vi "UpdateFeatureStudio.vi"(0 "Device In":T1, 5 "FeatureScript":string, 11 "error in":errorcluster) -> (4 "Device Out":T1, 6 "Comm":T2, 15 "error out":errorcluster)   [LabVIEW 2019]
uses:
  <userlib>/IoT Devices/_subVIs/HTTPComm.ctl
  <userlib>/Onshape/_SubVI/Cluster.ctl
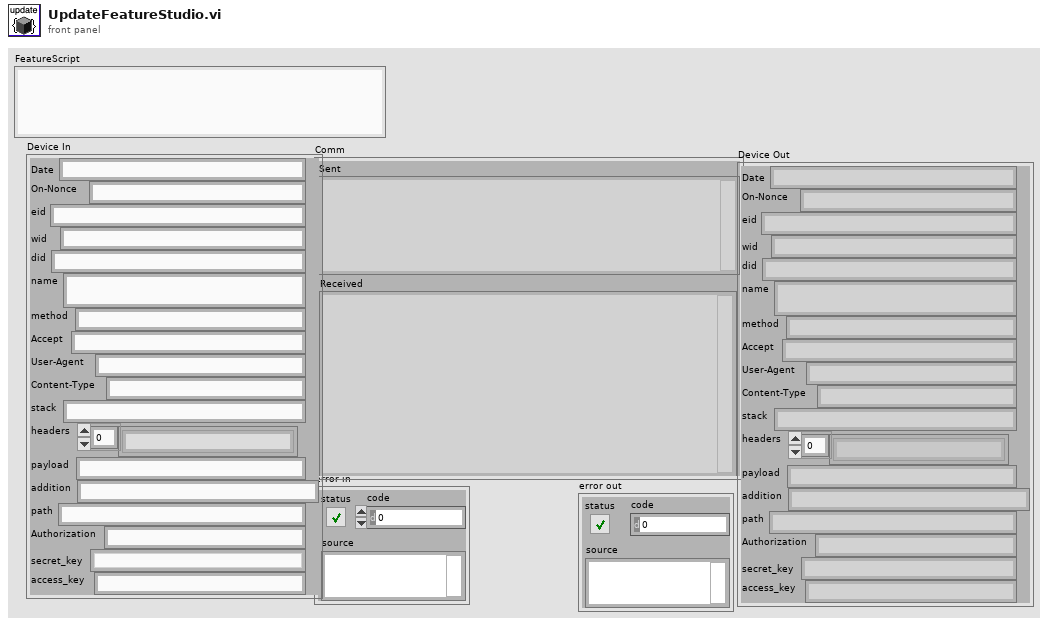
[diagram p1: front panel]
types:
  T1 = typedef "Cluster.ctl" = cluster{"Date":string, "On-Nonce":string, "eid":string, "wid":string, "did":string, "name":string, "method":string, "Accept":string, "User-Agent":string, "Content-Type":string, "stack":string, "headers":string[], "payload":string, "addition":string, "path":string, "Authorization":string, "secret_key":string, "access_key":string}
  T2 = typedef "HTTPComm.ctl" = cluster{"url":string, "sent headers":string, "sent body":string, "headers":string, "body":string, "Sent":string, "Received":string}
  T3 = cluster{"contents":string, "serializationVersion":string, "sourceMicroversion":string, "rejectMicroversionSkew":bool}
  T4 = cluster{"contents":string, "serializationVersion":string, "sourceMicroversion":string, "rejectMicroversionSkew":bool, "microversionSkew":bool, "libraryVersion":i32}
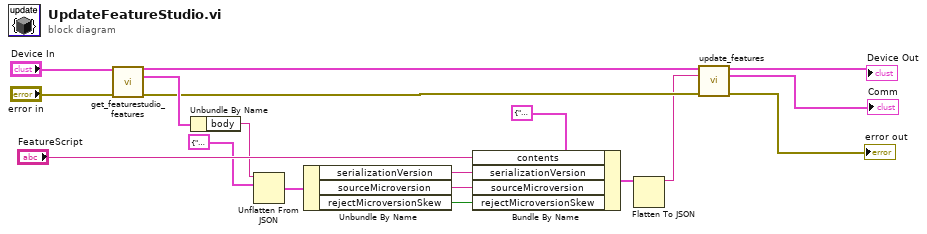
[diagram p0: block diagram]
diagram:
  n1 = call <userlib>:"get_featurestudio_features.vi"("Device In"="Device In", "Error in"="error in") -> ("Device Out"=w1:T1, "Comm"=w6:T2, "Error Out"=w5:errorcluster)  [unwired: 11 in]
  n2 = Unbundle By Name(w6) -> ("body"=w10:string)
  n3 = Unflatten From JSON(JSON string=w10, type and defaults=T4 {"contents"="", "serializationVersion"="", "sourceMicroversion"="", "rejectMicroversionSkew"=TRUE, "microversionSkew"=TRUE, "libraryVersion"=0}) -> (value=w14:T4)  [unwired: 5 in, 1 out]
  n4 = Unbundle By Name(w14) -> ("serializationVersion"=w15:string, "sourceMicroversion"=w16:string, "rejectMicroversionSkew"=w17:bool)
  n5 = Bundle By Name(cluster=T3 {"contents"="", "serializationVersion"="", "sourceMicroversion"="", "rejectMicroversionSkew"=TRUE}, "contents"="FeatureScript", "serializationVersion"=w15, "sourceMicroversion"=w16, "rejectMicroversionSkew"=w17) -> (w12:T3)
  n6 = Flatten To JSON(anything=w12) -> (JSON string=w2:string)  [unwired: 2 in, 1 out]
  n7 = call <userlib>:"update_features.vi"("Device In"=w1, "Features"=w2, "Error in"=w5) -> ("Device Out"=→"Device Out":T1, "Comm"=→"Comm":T2, "Error Out"=→"error out":errorcluster)  [unwired: 10 in]
